vi "Get Device Count.vi"(8 "error in (no error)":errorcluster) -> (0 "error out":errorcluster, 3 "Device Count":u32)   [LabVIEW 2016]
doc: "Gets the number of RTLSDR devices detected in the system."
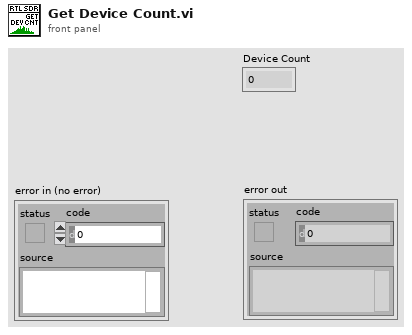
[diagram p1: front panel]
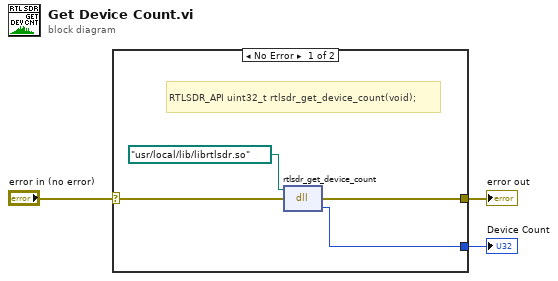
[diagram p0: block diagram]
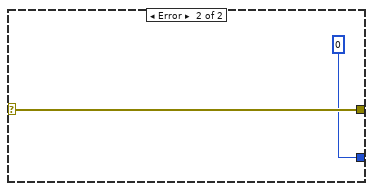
[diagram p2: hidden frame]
diagram:
  n1 = case shown="No Error" "error in (no error)" {
    selector: "error in (no error)" -> [w7 w9]
    tunnel: [w4 w9] -> w3
    tunnel: [w6 u32 0 ("return type")] -> w1
    frame No Error {
      # "RTLSDR_API uint32_t rtlsdr_get_device_count(void);"
      n2 = dll-call lib="C:/Program Files (x86)/National Instruments/LabVIEW 2016/user.lib/rtlsdr/rtlsdr.dll" fn="rtlsdr_get_device_count"(path in=path "/usr/local/lib/librtlsdr.so", error in=w7) -> (error out=w4:errorcluster, "return type"=w6:u32)  [unwired: 1 in, 1 out]
    }
    frame Error {
    }
  }
  "error out" <- w3
  "Device Count" <- w1
